vi "Create (Group Config).vi"(8 "error in (no error)":errorcluster, 10 "Group Config":refnum<class "Group Config.lvclass">) -> (0 "error out":errorcluster, 3 "Scaling out":refnum<class "Scaling.lvclass">)   [LabVIEW 2020, in "VolatusData.lvlib" / "Scaling.lvclass"]
uses:
  Scaling.lvclass
  VolatusConfig/Group/Group Config.lvclass
  Scaling.lvclass/Scaling.ctl
  VolatusConfig/Scaling/Scaling Config.lvclass
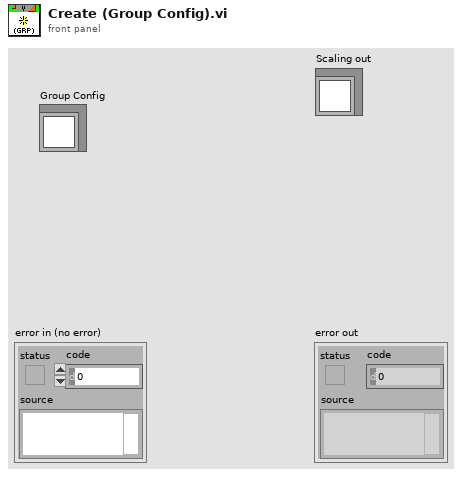
[diagram p1: front panel]
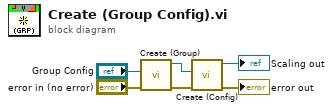
[diagram p0: block diagram]
diagram:
  n1 = call "Create (Group).vi"("error in (no error)"="error in (no error)", "Group Config"="Group Config") -> ("error out"=w4:errorcluster, "Scaling out"=w3:refnum<class "Scaling Config.lvclass">)  [unwired: 8 in]
  n2 = call "Create (Config).vi"("error in (no error)"=w4, "Scaling Config"=w3) -> ("error out"=→"error out":errorcluster, "VolatusScaling out"=→"Scaling out":refnum<class "Scaling.lvclass">)  [unwired: 8 in]
